vi "DSF.Engine.Plugin.Process Transfer.Parse.vi"(8 "error in (no error)":errorcluster, 9 "VS Channel Buffer in":dbl[](array[numeric]), 10 "Transfer":refnum<class "DSF.Engine.Transfer.lvclass">, 11 "Plugin in":refnum<class "Plugin.lvclass">) -> (0 "error out":errorcluster, 1 "VS Channel Buffer out":dbl[](array[numeric]), 3 "Plugin out":refnum<class "Plugin.lvclass">)   [LabVIEW 2016, in "DSF.Engine.lvlib" / "Plugin.lvclass"]
uses:
  Plugin.lvclass
  Transfer/DSF.Engine.Transfer.lvclass
  Transfer/DSF.Engine.Transfer.lvclass/DSF.Engine.Transfer.ctl
  Shared/Classes/Transfer/DSF.Shared.Configuration.Transfer.lvclass/DSF.Shared.Configuration.Transfer.ctl
  Buffer/DSF.Engine.Memory.Buffer.lvclass
  Shared/Classes/Transfer/DSF.Shared.Configuration.Transfer.lvclass
  Pointer/DSF.Engine.Pointer.DBL.lvclass
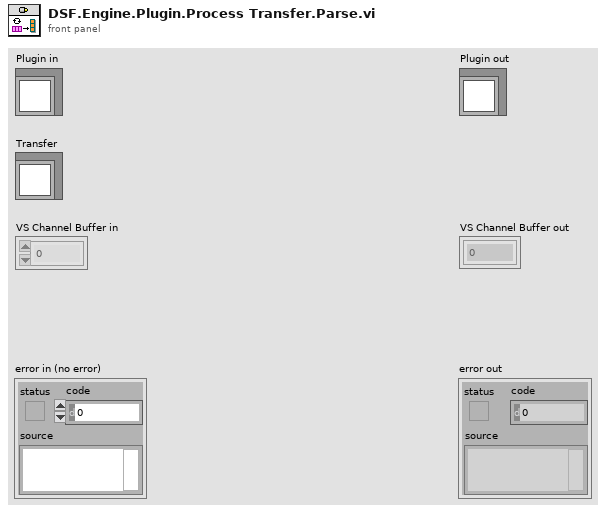
[diagram p1: front panel]
types:
  T1 = typedef "DSF.Shared.lvlib/DSF.Shared.Typedefs.Configuration.Transfer.Channel Block Descriptor.ctl" = cluster{"First Channel Descriptor":T2, "count":u64, "vs channel index":u64}
  T2 = typedef "DSF.Shared.lvlib/DSF.Shared.Typedefs.Configuration.Transfer.Channel Descriptor.ctl" = cluster{"Channel Parameters":T3, "VS Channel Ref":T5}
  T3 = typedef "DSF.Shared.lvlib/DSF.Shared.Typedefs.Configuration.Transfer.Channel Parameters.ctl" = cluster{"offset":u64, "data type":T4}
  T4 = typedef "DSF.Shared.lvlib/DSF.Shared.Typedefs.Data Type.ctl" = enum8{"Bool", "SGL", "DBL", "I8", "I16", "I32", "I64", "U8", "U16", "U32", "U64"}
  T5 = typedef "Custom Device API.lvlib/Custom Device Item Ref.ctl" = u64
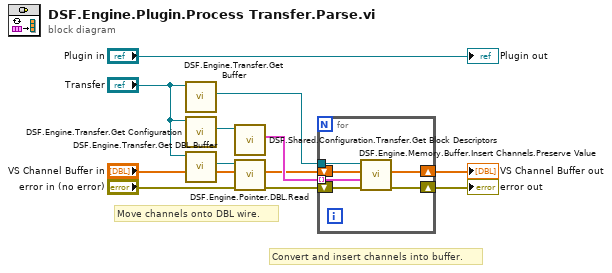
[diagram p0: block diagram]
diagram:
  # "Convert and insert channels into buffer."
  # "Move channels onto DBL wire."
  n1 = call "DSF.Engine.Transfer.Get Buffer.vi"("Transfer in"="Transfer") -> ("Buffer"=w8:refnum<class "DSF.Engine.Memory.Buffer.lvclass">)  [unwired: 9 in, 1 out]
  n2 = call "DSF.Engine.Transfer.Get Configuration.vi"("Transfer in"="Transfer") -> ("Configuration"=w12:refnum<class "DSF.Shared.Configuration.Transfer.lvclass">)  [unwired: 9 in, 1 out]
  n3 = call "DSF.Engine.Transfer.Get DBL Buffer.vi"("Transfer in"="Transfer") -> ("DBL Buffer"=w5:refnum<class "DSF.Engine.Pointer.DBL.lvclass">)  [unwired: 9 in, 1 out]
  n4 = call "DSF.Shared.Configuration.Transfer.Get Block Descriptors.vi"("Transfer Configuration in"=w12) -> ("Channel Blocks"=w7:T1[])  [unwired: 9 in, 1 out]
  n5 = call "DSF.Engine.Pointer.DBL.Read.vi"("error in (no error)"="error in (no error)", "buffer in"="VS Channel Buffer in", "DBL Pointer in"=w5) -> ("error out"=w1:errorcluster, "buffer out"=w2:dbl[])  [unwired: 6 in, 1 out]
  n6 = for {
    shift-right: [w16] -> w10
    shift-left: w2 -> [w17]
    shift-right: [w15] -> w11
    shift-left: w1 -> [w18]
    tunnel: w8 -> [w14]
    tunnel: w7 -> [w13] mode=indexing
    n7 = call "DSF.Engine.Memory.Buffer.Insert Channels.Preserve Value.vi"("error in (no error)"=w18, "Channel Block"=w13, "VS Channels Array in"=w17, "Buffer in"=w14) -> ("error out"=w15:errorcluster, "VS Channels Array out"=w16:dbl[])  [unwired: 5 in, 1 out]
  }
  "error out" <- w11
  "VS Channel Buffer out" <- w10
  "Plugin out" <- "Plugin in"
